vi "startNewLog.vi"(8 "error in (no error)":errorcluster, 11 "Logger in":refnum<class "Log.lvclass">) -> (0 "error out":errorcluster, 3 "Logger out":refnum<class "Log.lvclass">)   [LabVIEW 2013, in "Log.lvclass"]
uses:
  Log.lvclass
  Log.lvclass/Log.ctl
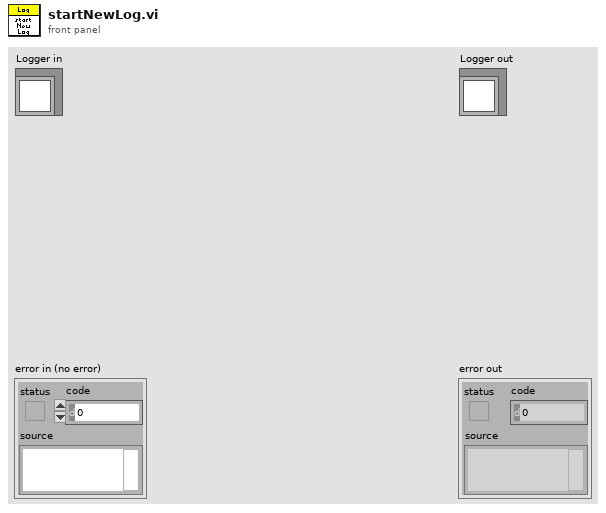
[diagram p1: front panel]
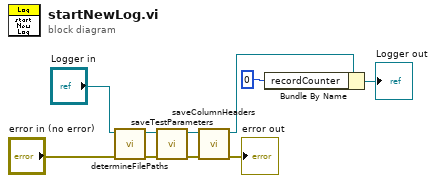
[diagram p0: block diagram]
diagram:
  n1 = call "determineFilePaths.vi"("error in (no error)"="error in (no error)", "Logger in"="Logger in") -> ("error out"=w2:errorcluster, "Logger out"=w1:refnum<class "Log.lvclass">)  [unwired: 8 in]
  n2 = call-dynamic "saveTestParameters.vi"("error in (no error)"=w2, "Logger in"=w1) -> ("error out"=w5:errorcluster, "Logger out"=w6:refnum<class "Log.lvclass">)  [unwired: 8 in]
  n3 = call "saveColumnHeaders.vi"("error in (no error)"=w5, "Logger in"=w6) -> ("error out"=→"error out":errorcluster, "Logger out"=w9:refnum<class "Log.lvclass">)  [unwired: 8 in]
  n4 = Bundle By Name(cluster=w9, "recordCounter"=u32 0) -> (→"Logger out":refnum<class "Log.lvclass">)
